vi "Old Reference Value.vi"(8 "error in (no error)":errorcluster, 11 "VISA resource name":refnum<visa-resource-name>) -> (0 "error out":errorcluster, 3 "VISA resource name out":refnum<visa-resource-name>)   [LabVIEW 2013, in "Fluke 5XXX Series Multicalibrators.lvlib"]
doc: "This VI sets the Calibrator output to the existing reference value and exit the error mode (if selected).\n\nNote:\n\nIf editing the output using FL5XMCAL Set Edit Field.vi and FL5XMCAL Change Output Value.vi and you want to return to the reference value, use this function. If editing the output and you want to make the edited value the new reference, use FL5XMCAL New Reference Value.vi."
uses:
  Fluke 5XXX Series Multicalibrators.lvlib
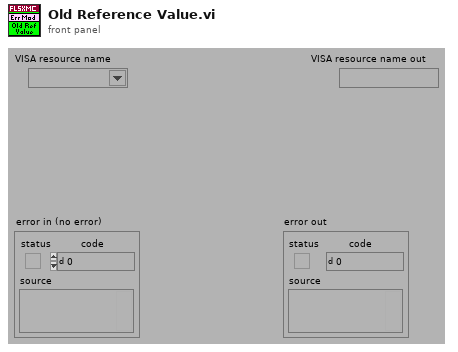
[diagram p1: front panel]
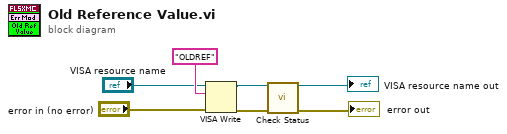
[diagram p0: block diagram]
diagram:
  n1 = VISA Write(VISA resource name="VISA resource name", write buffer="OLDREF", error in (no error)="error in (no error)") -> (VISA resource name out=w5:refnum<visa-resource-name>, error out=w6:errorcluster)  [unwired: 1 out]
  n2 = call "Check Status.vi"("VISA resource name"=w5, "error in (no error)"=w6) -> ("VISA resource name out"=→"VISA resource name out":refnum<visa-resource-name>, "error out"=→"error out":errorcluster)  [unwired: 12 in]
